vi "rad_View App Image Info.vi"(11 "App Images Information":T1) -> ()   [LabVIEW 2020]
uses:
  TypeDefs/rad_AppImage Information.ctl
  TypeDefs/rad_Application Image Properties.ctl
  TypeDefs/rad_FPGA Properties.ctl
  TypeDefs/rad_FPGA Flash Properties.ctl
  <vilib>/Utility/miscctls.llb/LVRowAndColumnTypeDef.ctl
  <vilib>/Utility/miscctls.llb/LVRowAndColumnUnsignedTypeDef.ctl
panel:
  in  "Image Information":i32(listbox)
  out "error out":errorcluster
  in  "error in (no error)":errorcluster
  in  "ViewInstalledSoftware":bool
  in  "Close":bool
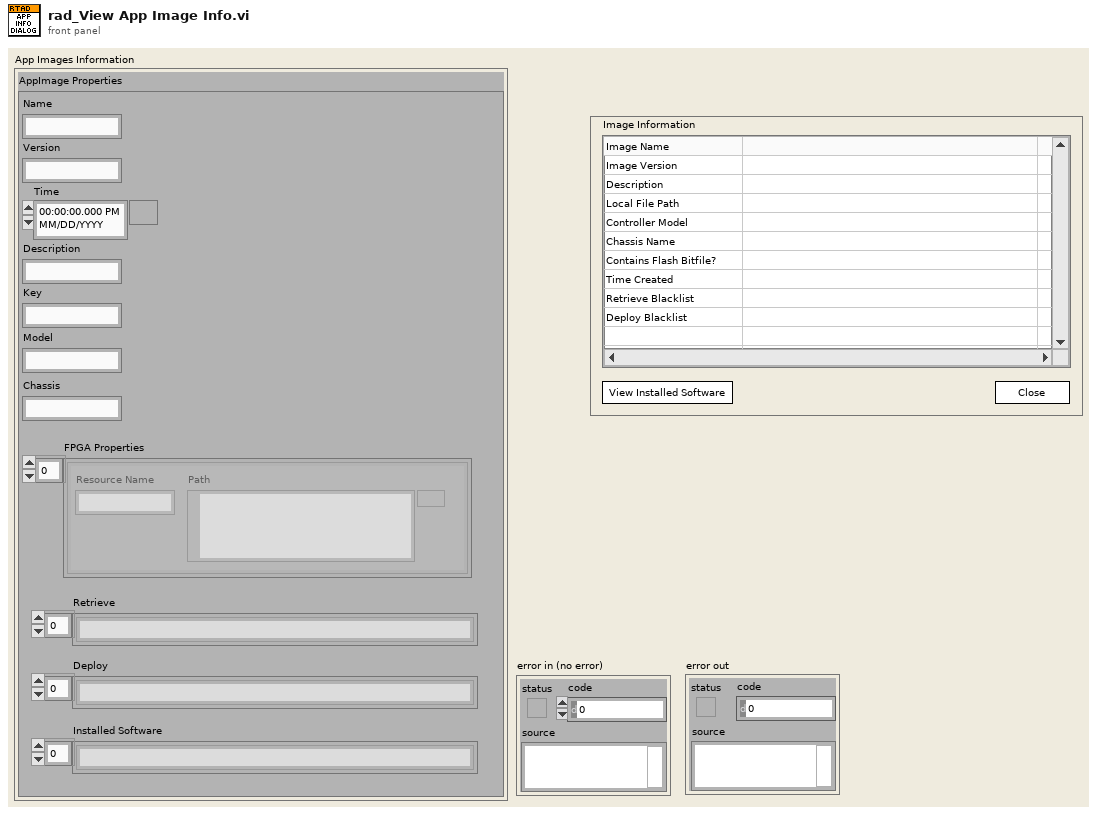
[diagram p1: front panel]
types:
  T1 = typedef "rad_AppImage Information.ctl" = cluster{"AppImage Properties":T2, "AppImage Path":path}
  T2 = typedef "rad_Application Image Properties.ctl" = cluster{"Name":string, "Version":string, "Time":timestamp, "Description":string, "Key":string, "Chassis":string, "FPGA Properties":T3, "Model":string, "Retrieve":string[], "Deploy":string[], "Installed Software":string[]}
  T3 = typedef "rad_FPGA Properties.ctl" = T4[]
  T4 = typedef "rad_FPGA Flash Properties.ctl" = cluster{"Resource Name":string, "Path":path}
  T5 = typedef "LVRowAndColumnUnsignedTypeDef.ctl" = cluster{"Row":u32, "Column":u32}
  T6 = typedef "LVRowAndColumnTypeDef.ctl" = cluster{"Row":i32, "Column":i32}
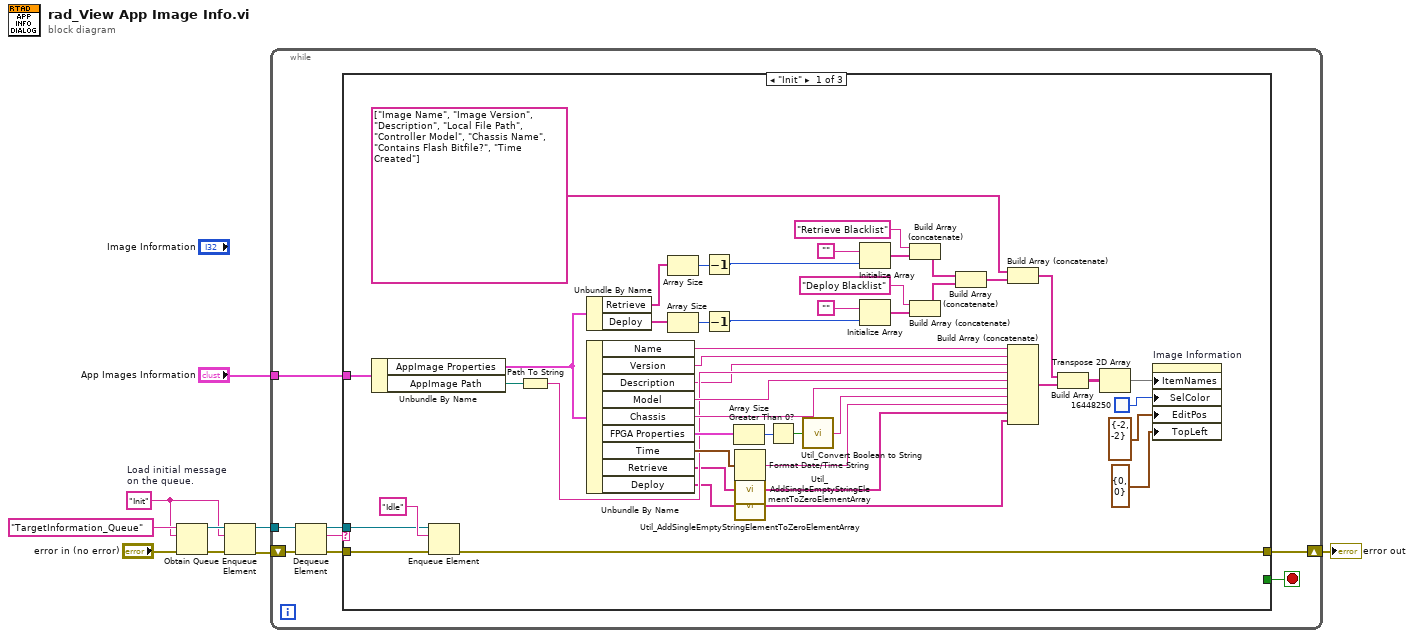
[diagram p0: block diagram]
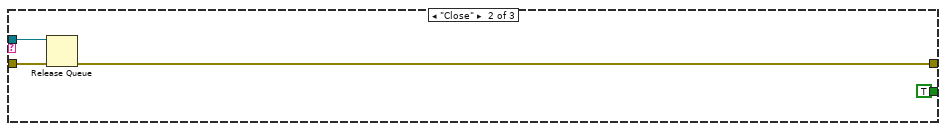
[diagram p2: hidden frame]
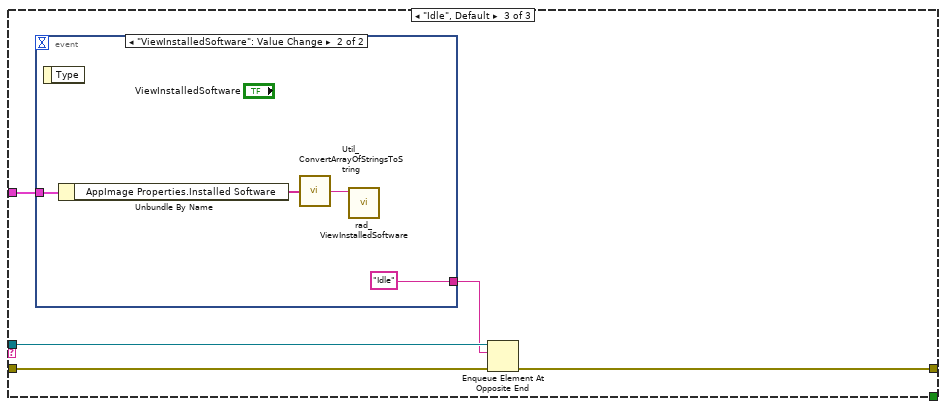
[diagram p3: hidden frame]
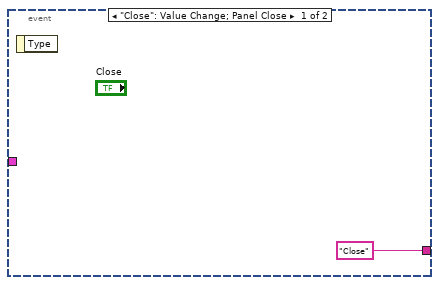
[diagram p4: hidden frame]
diagram:
  w2 = "Init"  # Load initial message on the queue.
  n1 = Obtain Queue(name (unnamed)="TargetInformation_Queue" ("Message Queue Name"), element data type=w2, error in (no error)="error in (no error)") -> (queue out=w7:refnum<queue>, error out=w4:errorcluster)  [unwired: 2 in, 1 out]
  n2 = Enqueue Element(queue=w7, element=w2, error in (no error)=w4) -> (queue out=w5:refnum<queue>, error out=w3:errorcluster)  [unwired: 1 in, 1 out]
  n3 = while {
    shift-right: [w13] -> w1
    shift-left: w3 -> [w11]
    tunnel: "App Images Information" -> [w10]
    tunnel: w5 -> [w17]
    stop <- w12 stop-if-true
    n4 = Dequeue Element(queue=w17, error in (no error)=w11) -> (queue out=w15:refnum<queue>, element=w16:string, error out=w14:errorcluster)  [unwired: 1 in, 1 out]
    n5 = case shown="\"Init\"" w16 {
      tunnel: w15 -> [w60 w65 w70]
      tunnel: w14 -> [w61 w66 w69]
      tunnel: [w59 w64 w71] -> w13
      tunnel: [_ TRUE _] -> w12
      tunnel: w10 -> [w63 _ w72]
      frame "Init" {
        n6 = Unbundle By Name(w63) -> ("AppImage Properties"=w56:T2, "AppImage Path"=w33:path)
        n7 = Enqueue Element(queue=w60, element="Idle" ("Message Name"), error in (no error)=w61) -> (error out=w59:errorcluster)  [unwired: 1 in, 2 out]
        n8 = Path To String(path=w33) -> (string=w34:string)
        n9 = Unbundle By Name(w56) -> ("Retrieve"=w57:string[], "Deploy"=w58:string[])
        n10 = Unbundle By Name(w56) -> ("Name"=w29:string, "Version"=w30:string, "Description"=w32:string, "Model"=w39:string, "Chassis"=w40:string, "FPGA Properties"=w41:T3, "Time"=w42:timestamp, "Retrieve"=w21:string[], "Deploy"=w19:string[])
        n11 = Array Size(array=w57) -> (size(s)=w44:i32)
        n12 = Array Size(array=w58) -> (size(s)=w48:i32)
        n13 = Decrement(x=w44) -> (x-1=w23:i32)
        n14 = Decrement(x=w48) -> (x-1=w22:i32)
        n15 = Array Size(array=w41) -> (size(s)=w35:i32)
        n16 = Format Date/Time String(seconds (now)=w42) -> (date/time string=w38:string)  [unwired: 2 in]
        n17 = call "Util_AddSingleEmptyStringElementToZeroElementArray.vi"("Array In"=w21) -> ("Array Out"=w20:string[])
        n18 = call "Util_AddSingleEmptyStringElementToZeroElementArray.vi"("Array In"=w19) -> ("Array Out"=w18:string[])
        n19 = Greater Than 0?(x=w35) -> (x > 0?=w36:bool)
        n20 = call "Util_Convert Boolean to String.vi"("Boolean"=w36) -> ("String"=w37:string)  [unwired: 4 out]
        n21 = Initialize Array("", w23) -> (w45:string[])
        n22 = Initialize Array("", w22) -> (w47:string[])
        n23 = Build Array (concatenate)("Retrieve Blacklist", w45) -> (w51:string[])
        n24 = Build Array (concatenate)("Deploy Blacklist", w47) -> (w52:string[])
        n25 = Build Array (concatenate)(w51, w52) -> (w53:string[])
        n26 = Build Array (concatenate)(string[] ["Image Name", "Image Version", "Description", "Local File Path", "Controller Model", "Chassis Name", "Contains Flash Bitfile?", "Time Created"] ("element"), w53) -> (w55:string[])
        n27 = Build Array (concatenate)(w29, w30, w32, w34, w39, w40, w37, w38, w20, w18) -> (w31:string[])
        n28 = Build Array(w55, w31) -> (w28:string[][])
        n29 = Transpose 2D Array(2D array=w28) -> (transposed array=w27:string[][])
        n30 = property on="Image Information" class="MCListbox (strict)"("ItemNames"=w27, "SelColor"=u32 16448250, "EditPos"=T6 {"Row"=-2, "Column"=-2} ("Edit Position"), "TopLeft"=T5 {"Row"=0, "Column"=0} ("Top Left Visible Cell")) -> ()  [unwired: 2 in, 2 out]
      }
      frame "Close" {
        n31 = Release Queue(queue=w65, error in (no error)=w66) -> (error out=w64:errorcluster)  [unwired: 1 in, 2 out]
      }
      frame "Idle", Default {
        n32 = event shown="[1] \"ViewInstalledSoftware\": Value Change" {
          selector: _ -> [_ _]
          dyn-events: _ -> [_ _]
          timeout: _ -> [_ _]
          tunnel: w72 -> [_ w77]
          tunnel: ["Close" ("Message Name") "Idle" ("Message Name")] -> w68
          event "Close": Value Change; Panel Close {
            n33 = event-data() -> ()  [unwired: 1 in, 1 out]
          }
          event "ViewInstalledSoftware": Value Change {
            n34 = event-data() -> ()  [unwired: 1 in, 1 out]
            n35 = Unbundle By Name(w77) -> ("AppImage Properties.Installed Software"=w76:string[])
            n36 = call "Util_ConvertArrayOfStringsToString.vi"("Array<string>"=w76) -> ("String"=w75:string)
            n37 = call "rad_ViewInstalledSoftware.vi"("Installed Software"=w75) -> ()  [unwired: 11 in]
          }
        }
        n38 = Enqueue Element At Opposite End(queue=w70, element=w68, error in (no error)=w69) -> (error out=w71:errorcluster)  [unwired: 1 in, 2 out]
      }
    }
  }
  "error out" <- w1
